vi "(auto) SAVE.vi"(0 "I2C Ref Out in":T7, 1 "CurDot":i32, 2 "Angles":dbl[](array[numeric]), 3 "Left_enc":i32[](array[numeric]), 4 "Right_enc":i32[](array[numeric]), 5 "M_enc":i32[](array[numeric]), 6 "G_enc":i32[](array[numeric]), 7 "error in (no error)":errorcluster, 9 "L_enc In":T1, 11 "R_enc In":T1, 15 "M_enc In":T1, 17 "G_enc In":T1) -> (20 "I2C Ref Out out":T7, 22 "Angles out":dbl[](array[numeric]), 23 "Left_enc out":i32[](array[numeric]), 24 "Right_enc out":i32[](array[numeric]), 25 "M_enc out":i32[](array[numeric]), 26 "G_enc out":i32[](array[numeric]), 27 "error out":errorcluster)   [LabVIEW 2017]
uses:
  <vilib>/myRIO/Instrument Drivers/Onboard IO/I2C/typedefs/I2C Reference.ctl
  <vilib>/myRIO/Common/Instrument Driver Framework/Utilities/typedefs/myRIO Generic Hardware Reference.ctl
  <vilib>/myRIO/Common/Instrument Driver Framework/Utilities/typedefs/Hardware Version Enum.ctl
  <vilib>/myRIO/Common/Instrument Driver Framework/Utilities/typedefs/myRIO v1.0 Reference.ctl
  <vilib>/myRIO/Common/Instrument Driver Framework/Utilities/typedefs/Generic FPGA Reference.ctl
  <vilib>/myRIO/Common/Instrument Driver Framework/myRIO v1.0/I2C/typedefs/I2C Channels Enum.ctl
  <vilib>/myRIO/Instrument Drivers/Onboard IO/I2C/typedefs/I2C Configuration.ctl
  <vilib>/myRIO/Instrument Drivers/Onboard IO/I2C/typedefs/I2C Transfer Rate.ctl
  <vilib>/myRIO/Instrument Drivers/Onboard IO/Encoder/typedefs/Encoder Reference.ctl
  <vilib>/myRIO/Common/Instrument Driver Framework/myRIO v1.0/Encoder/typedefs/Encoder Channels Enum.ctl
  <vilib>/Utility/error.llb/Error Cluster From Error Code.vi
  <vilib>/myRIO/Common/Instrument Driver Framework/myRIO v1.0/Encoder/vis/myRIO v1.0 Read Encoder.vi
  <vilib>/myRIO/Instrument Drivers/Onboard IO/Encoder/Encoder.lvlib
  <vilib>/myRIO/Instrument Drivers/Onboard IO/I2C/I2C.lvlib
panel:
  out "G_enc Out":T1
  out "M_enc Out":T1
  out "R_enc Out":T1
  out "L_enc Out":T1
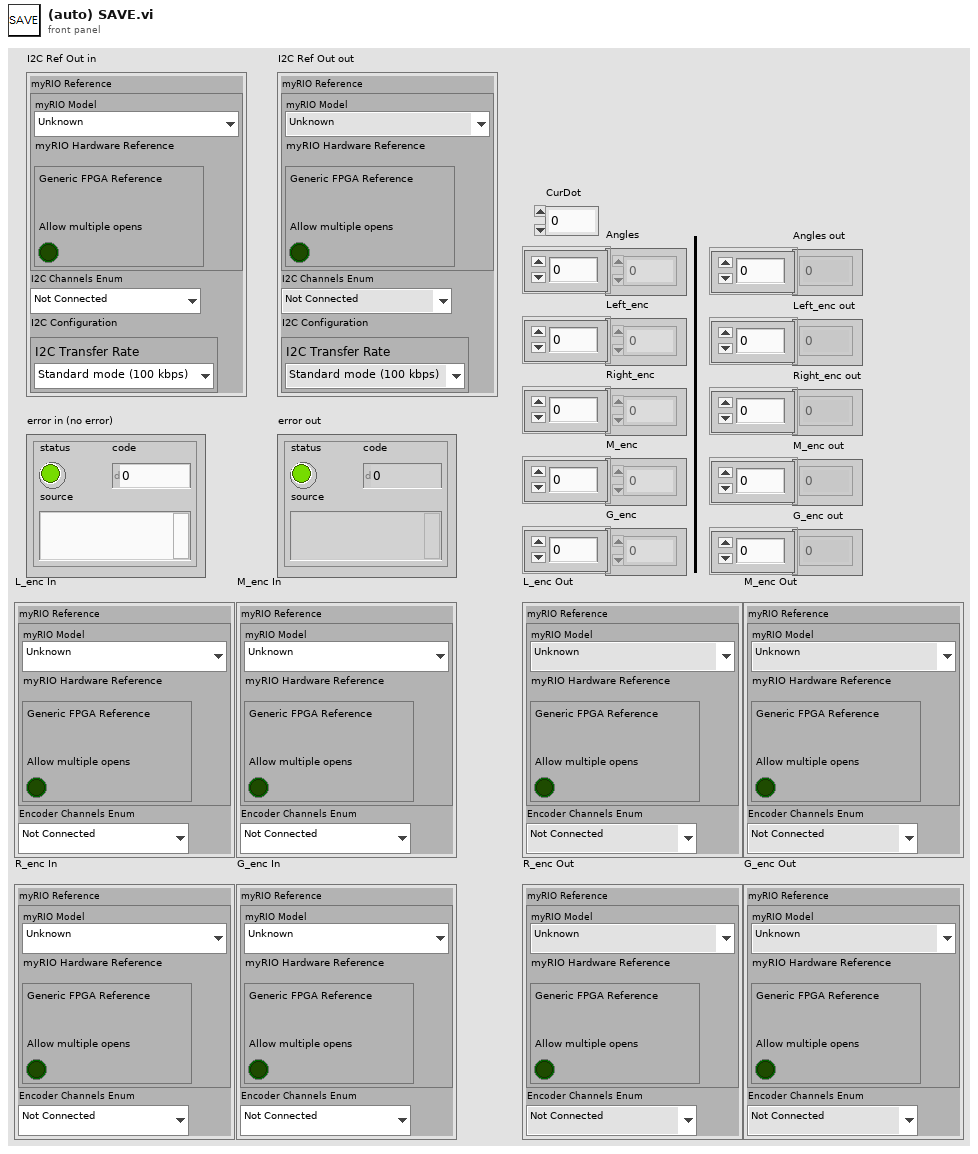
[diagram p1: front panel]
types:
  T1 = typedef "Encoder.lvlib/Encoder Reference.ctl" = cluster{"myRIO Reference":T2, "Encoder Channels Enum":T6}
  T2 = typedef "myRIO Generic Hardware Reference.ctl" = cluster{"myRIO Model":T3, "myRIO Hardware Reference":T4}
  T3 = typedef "Hardware Version Enum.ctl" = enum16{"Unknown", "myRIO-1900", "myRIO-1950", "roboRIO", "NI ELVIS RIO CM"}
  T4 = typedef "myRIO v1.0 Reference.ctl" = cluster{"Generic FPGA Reference":T5, "Allow multiple opens":bool}
  T5 = typedef "Generic FPGA Reference.ctl" = refnum<k20>
  T6 = typedef "Encoder Channels Enum.ctl" = enum16{"Not Connected", "C/ENC0", "C/ENC1", "A/ENC", "B/ENC", "DIO/ENC0", "DIO/ENC1", "DIO/ENC2", "DIO/ENC3", "DIO/ENC4"}
  T7 = typedef "I2C.lvlib/I2C Reference.ctl" = cluster{"myRIO Reference":T2, "I2C Channels Enum":T8, "I2C Configuration":T9}
  T8 = typedef "I2C Channels Enum.ctl" = enum16{"Not Connected", "A/I2C", "B/I2C", "I2C/I2C"}
  T9 = typedef "I2C.lvlib/I2C Configuration.ctl" = cluster{"I2C Transfer Rate":T10}
  T10 = typedef "I2C.lvlib/I2C Transfer Rate.ctl" = enum16{"Standard mode (100 kbps)", "Fast mode (400 kbps)"}
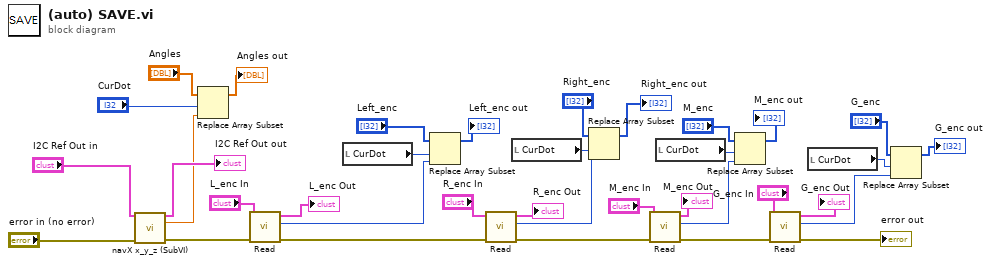
[diagram p0: block diagram]
diagram:
  n1 = call "navX x_y_z (SubVI).vi"("I2C Ref Out in"="I2C Ref Out in", "error in (no error)"="error in (no error)") -> ("I2C Ref Out out"=→"I2C Ref Out out":T7, "value Z"=w29:ext, "error out"=w28:errorcluster)  [unwired: 9 in, 2 out]
  n2 = Replace Array Subset(array="Angles", new element=w29, index="CurDot") -> (→"Angles out":dbl[])
  n3 = call <vilib>:"Read.vi"("error in (no error)"=w28, "Encoder Ref In"="L_enc In") -> ("error out"=w19:errorcluster, "Counter Value"=w22:i32, "Encoder Ref Out"=→"L_enc Out":T1)  [unwired: 5 in, 2 out]
  n4 = local read "CurDot"() -> (w25:i32)
  n5 = Replace Array Subset(array="Left_enc", new element=w22, index=w25) -> (→"Left_enc out":i32[])
  n6 = call <vilib>:"Read.vi"("error in (no error)"=w19, "Encoder Ref In"="R_enc In") -> ("error out"=w14:errorcluster, "Counter Value"=w15:i32, "Encoder Ref Out"=→"R_enc Out":T1)  [unwired: 5 in, 2 out]
  n7 = local read "CurDot"() -> (w16:i32)
  n8 = Replace Array Subset(array="Right_enc", new element=w15, index=w16) -> (→"Right_enc out":i32[])
  n9 = call <vilib>:"Read.vi"("error in (no error)"=w14, "Encoder Ref In"="M_enc In") -> ("error out"=w7:errorcluster, "Counter Value"=w11:i32, "Encoder Ref Out"=→"M_enc Out":T1)  [unwired: 5 in, 2 out]
  "error out" <- w7
  n10 = local read "CurDot"() -> (w10:i32)
  n11 = Replace Array Subset(array="M_enc", new element=w11, index=w10) -> (→"M_enc out":i32[])
  n12 = call <vilib>:"Read.vi"("error in (no error)"=w7, "Encoder Ref In"="G_enc In") -> ("Counter Value"=w4:i32, "Encoder Ref Out"=→"G_enc Out":T1)  [unwired: 5 in, 3 out]
  n13 = local read "CurDot"() -> (w1:i32)
  n14 = Replace Array Subset(array="G_enc", new element=w4, index=w1) -> (→"G_enc out":i32[])
